vi "TC_to_DSC.vi"(7 "Enum":enum16{"CF", "MNK"}(ring)=enum."MNK", 9 "I":dbl[](array[numeric]), 10 "T":dbl[](array[numeric]), 11 "R":dbl[](array[numeric])) -> ()   [LabVIEW 2013]
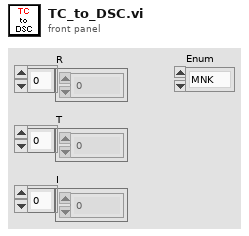
[diagram p1: front panel]
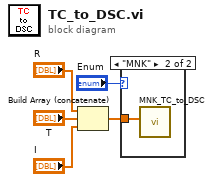
[diagram p0: block diagram]
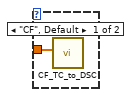
[diagram p2: hidden frame]
diagram:
  n1 = Build Array (concatenate)("R", "T", "I") -> (w5:dbl[])
  n2 = case shown="\"MNK\"" "Enum" {
    tunnel: w5 -> [w6 w7]
    frame "CF", Default {
      n3 = call "CF_TC_to_DSC.vi"("dbl"=w6) -> ()  [unwired: 3 in]
    }
    frame "MNK" {
      n4 = call "MNK_TC_to_DSC.vi"("dbl"=w7) -> ()  [unwired: 3 in]
    }
  }
